vi "ClassPanel.vi"(8 "error in (no error)":errorcluster caption="entrée d'erreur (pas d'erreur)", 11 "Device.lvclass":refnum<class "BaseDevice.lvclass">) -> (0 "error out":errorcluster caption="sortie d'erreur", 3 "Device.lvclass Out":refnum<class "BaseDevice.lvclass">)   [LabVIEW 2010, in "BaseDevice.lvclass"]
uses:
  BaseDevice.lvclass
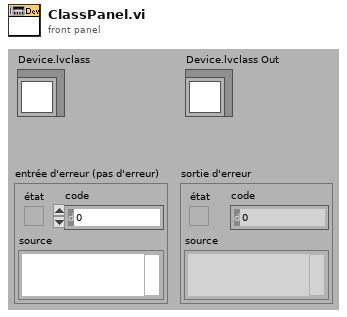
[diagram p1: front panel]
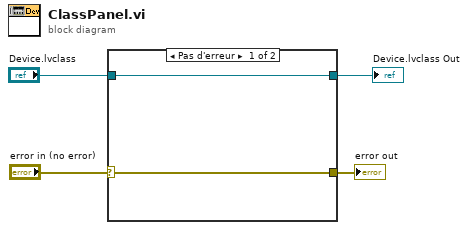
[diagram p0: block diagram]
diagram:
  n1 = case shown="Pas d'erreur" "error in (no error)" {
    selector: "error in (no error)" -> [w5 w7]
    tunnel: [w6 w8] -> w4
    tunnel: "Device.lvclass" -> [w6 w8]
    tunnel: [w5 w7] -> w1
    frame No Error {
    }
    frame Error {
    }
  }
  "error out" <- w1
  "Device.lvclass Out" <- w4
